vi "QuickFWCopy.vi"(8 "Error In":errorcluster, 10 "Override lib path?":bool, 11 "Arduino lib directory":path=path "C:/Users/chris/Documents/Arduino/libraries") -> (0 "Error Out":errorcluster)   [LabVIEW 2019, in "LINXx.lvlib"]
doc: "Dev helper to copy firmware to build directory. Defaults to local PlatformIO project in repo root."
uses:
  LINXx.lvlib
  <vilib>/MakerHub/LINX/Private/Type Defs/Firmware Library Component.ctl
  <vilib>/Utility/config.llb/Read Key (String).vi
  <vilib>/Utility/config.llb/NI_LVConfig.lvlib
  <vilib>/MakerHub/Toolbox/LMH-Toolbox.lvlib
  <vilib>/MakerHub/LINX/LMH-LINX.lvlib
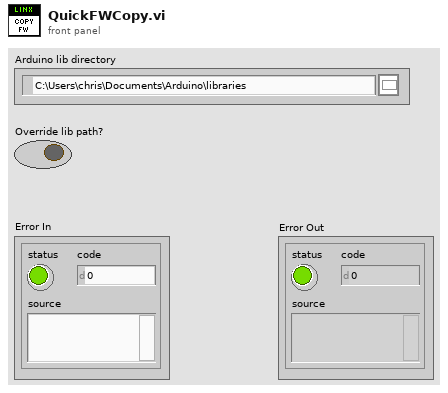
[diagram p1: front panel]
types:
  T1 = typedef "NI_LVConfig.lvlib/Config Data RefNum.ctl" = refnum<k1>
  T2 = typedef "LMH-LINX.lvlib/Firmware Library Component.ctl" = cluster{"Source":path, "Destination":path}
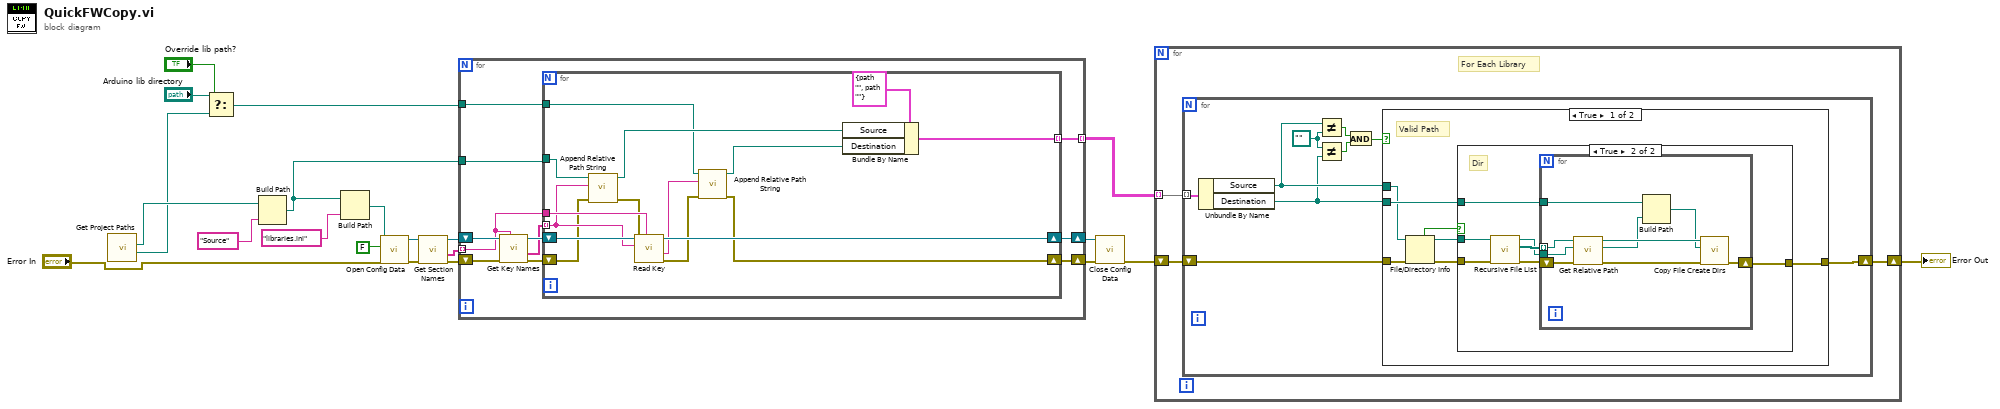
[diagram p0: block diagram]
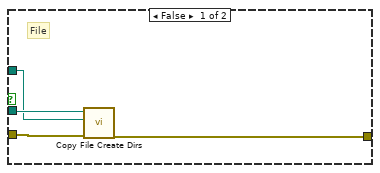
[diagram p2: hidden frame]
diagram:
  n1 = call "Get Project Paths.vi"() -> ("PlatformIO lib path"=w4:path, "Firmware path"=w6:path)  [unwired: 9 in, 1 out]
  n2 = Select(t="Arduino lib directory", s="Override lib path?", f=w4) -> (s? t:f=w5:path)
  n3 = Build Path(base path=w6, name or relative path="Source") -> (appended path=w7:path)
  n4 = Build Path(base path=w7, name or relative path="libraries.ini") -> (appended path=w10:path)
  n5 = call <vilib>:"Open Config Data.vi"("error in (no error)"="Error In", "create file if necessary (T)"=FALSE, "configuration file path"=w10) -> ("error out"=w20:errorcluster, "refnum"=w21:T1)  [unwired: 6 in, 1 out]
  n6 = call <vilib>:"Get Section Names.vi"("error in (no error)"=w20, "refnum"=w21) -> ("error out"=w16:errorcluster, "section names"=w14:string[], "refnum out"=w18:T1)  [unwired: 7 in]
  n7 = for {
    shift-right: [w29] -> w17
    shift-left: w18 -> [w32]
    shift-right: [w27] -> w15
    shift-left: w16 -> [w31]
    tunnel: w14 -> [w25] mode=indexing
    tunnel: w7 -> [w24]
    tunnel: [w23] -> w13 mode=indexing
    tunnel: w5 -> [w22]
    n8 = call <vilib>:"Get Key Names.vi"("section"=w25, "error in (no error)"=w31, "refnum"=w32) -> ("error out"=w28:errorcluster, "key names"=w26:string[], "refnum out"=w30:T1)  [unwired: 5 in, 1 out]
    n9 = for {
      shift-right: [w46] -> w29
      shift-left: w30 -> [w47]
      shift-right: [w37] -> w27
      shift-left: w28 -> [w39]
      tunnel: w26 -> [w40] mode=indexing
      tunnel: w25 -> [w45]
      tunnel: w24 -> [w41]
      tunnel: [w34] -> w23 mode=indexing
      tunnel: w22 -> [w33]
      n10 = call <vilib>:"Append Relative Path String.vi"("Error In"=w39, "Relative Path"=w40, "Base Path"=w41) -> ("Error Out"=w38:errorcluster, "Absolute Path"=w36:path)  [unwired: 7 in]
      n11 = call-poly <vilib>:"Read Key.vi"("section"=w45, "error in (no error)"=w38, "key"=w40, "refnum"=w47) -> ("error out"=w44:errorcluster, "value"=w43:string, "refnum out"=w46:T1)  [unwired: 4 in, 1 out]
      n12 = call <vilib>:"Append Relative Path String.vi"("Error In"=w44, "Relative Path"=w43, "Base Path"=w33) -> ("Error Out"=w37:errorcluster, "Absolute Path"=w35:path)  [unwired: 7 in]
      n13 = Bundle By Name(cluster=T2 {"Source"=path "", "Destination"=path ""} ("Library Component"), "Source"=w36, "Destination"=w35) -> (w34:T2)
    }
  }
  n14 = call <vilib>:"Close Config Data.vi"("error in (no error)"=w15, "refnum"=w17) -> ("error out"=w12:errorcluster)  [unwired: 8 in, 1 out]
  n15 = for {
    tunnel: w13 -> [w49] mode=indexing
    shift-right: [w48] -> w11
    shift-left: w12 -> [w50]
    # "For Each Library"
    n16 = for {
      tunnel: w49 -> [w59] mode=indexing
      shift-right: [w58] -> w48
      shift-left: w50 -> [w51]
      w55 = path ""
      n17 = Unbundle By Name(w59) -> ("Source"=w54:path, "Destination"=w53:path)
      n18 = Not Equal?(x=w54, y=w55) -> (x != y?=w57:bool)
      n19 = Not Equal?(x=w55, y=w53) -> (x != y?=w56:bool)
      n20 = And(x=w57, y=w56) -> (x .and. y?=w52:bool)
      n21 = case shown="True" w52 {
        tunnel: [w65 w87] -> w58
        tunnel: w53 -> [w66 _]
        tunnel: w54 -> [w63 _]
        tunnel: w51 -> [w64 w87]
        frame True {
          # "Valid Path"
          n22 = File/Directory Info(path=w63, error in=w64) -> (path out=w62:path, directory=w60:bool, error out=w61:errorcluster)  [unwired: 4 out]
          n23 = case shown="True" w60 {
            tunnel: w66 -> [w68 w74]
            tunnel: [w67 w73] -> w65
            tunnel: w62 -> [w69 w72]
            tunnel: w61 -> [w70 w71]
            frame False {
              # "File"
              n24 = call <vilib>:"Copy File Create Dirs.vi"("Error In"=w70, "Destination"=w68, "Source"=w69) -> ("Error Out"=w67:errorcluster)  [unwired: 8 in]
            }
            frame True {
              # "Dir"
              n25 = call <vilib>:"Recursive File List.vi"("error in (no error)"=w71, "Folder Path"=w72) -> ("error out"=w77:errorcluster, "All Files in Dir"=w76:path[], "dup Folder Path"=w75:path)  [unwired: 5 in, 2 out]
              n26 = for {
                tunnel: w76 -> [w85] mode=indexing
                tunnel: w75 -> [w84]
                tunnel: w74 -> [w81]
                shift-right: [w78] -> w73
                shift-left: w77 -> [w86]
                n27 = call <vilib>:"Get Relative Path.vi"("Error In"=w86, "Relative Path Root"=w84, "File / Folder"=w85) -> ("Error Out"=w83:errorcluster, "Relative Path"=w80:path, "Duplicate File / Folder"=w82:path)  [unwired: 6 in]
                n28 = Build Path(base path=w81, name or relative path=w80) -> (appended path=w79:path)
                n29 = call <vilib>:"Copy File Create Dirs.vi"("Error In"=w83, "Destination"=w79, "Source"=w82) -> ("Error Out"=w78:errorcluster)  [unwired: 8 in]
              }
            }
          }
        }
        frame False {
          # "Invalid Path"
        }
      }
    }
  }
  "Error Out" <- w11
